vi "Part 1.vi"(11 "Input":string="#############\n#...........#\n###B#C#A#B###\n  #D#C#B#A#\n  #D#B#A#C#\n  #C#D#D#A#\n  #########") -> (3 "Output":i64=49742)   [LabVIEW 2020]
panel:
  out "Moves":string[](array[string])=["H0 -> C0", "H10 -> B0", "H9 -> B1", "H7 -> C1", "H1 -> C2", "H5 -> B2", "H3 -> B3", "H5 -> B3", "H7 -> B2", "H7 -> D0", "H7 -> B1", "H5 -> C3", "H9 -> C3", "H10 -> C2", "H10 -> D1", "H7 -> D2", "H7 -> C1", "H9 -> D3", "H5 -> D3", "H3 -> D2", "H3 -> A0", "H3 -> B0", "H7 -> A1", "H7 -> D1", "H7 -> A2", "H7 -> D0", "H5 -> A3", "H1 -> A3", "H5 -> C0", "H9 -> A2", "H10 -> A1", "H0 -> A0"]
  out "Lowest":i64=49742
  out "Solved":i32=137
  out "Paths":i32=60
  out "Counter":i32=1143083
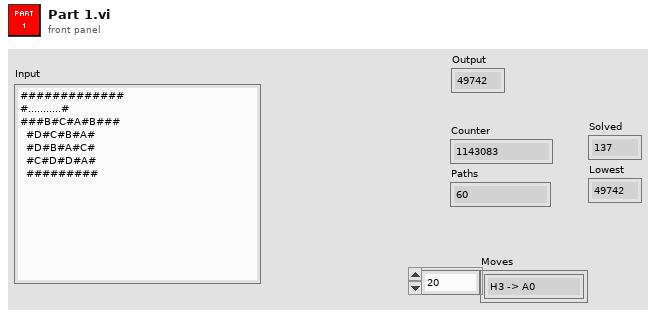
[diagram p1: front panel]
types:
  T1 = typedef "Data.ctl" = cluster{"Score":i64, "Data":cluster{"Hallway":string[], "Column A":string[], "Column B":string[], "Column C":string[], "Column D":string[]}, "Solved":bool, "Moves":string[]}
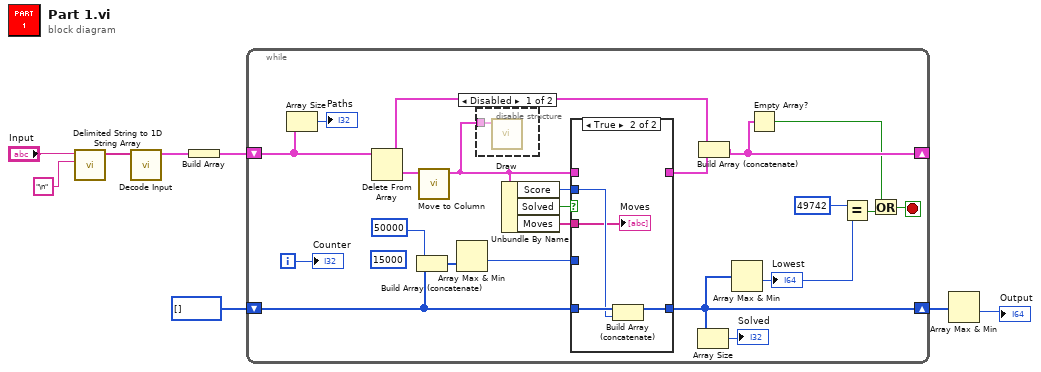
[diagram p0: block diagram]
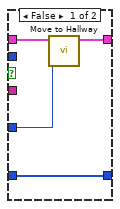
[diagram p3: hidden frame]
diagram:
  n1 = call <vilib>:"Delimited String to 1D String Array.vi"("delimiter"="\n", "delimited string"="Input") -> ("string array"=w6:string[])  [unwired: 9 in]
  n2 = call "Decode Input.vi"("Input"=w6) -> ("Data"=w1:T1)  [unwired: 10 in]
  n3 = Build Array(w1) -> (w5:T1[])
  n4 = while {
    shift-right: [w24] -> _
    shift-left: w5 -> [w18]
    shift-right: [w22] -> w3
    shift-left: i64[] [] -> [w21]
    i -> [w30]
    stop <- w10 stop-if-true
    (unwired) i64 15000 ("Max Score")
    n5 = Array Size(array=w18) -> (size(s)=→"Paths":i32)
    n6 = Delete From Array(array=w18) -> (deleted portion=w17:T1, array with subset deleted=w26:T1[])  [unwired: 2 in]
    n7 = Build Array (concatenate)(i64 50000 ("Max Score"), w21) -> (w20:i64[])
    n8 = call "Move to Column.vi"("Data In"=w17) -> ("Data Out"=w16:T1)  [unwired: 10 in]
    n9 = Array Max & Min(array=w20) -> (min value=w19:i64)  [unwired: 3 out]
    n10 = disable-structure shown="Disabled" {
      disable-tunnel: w16 -> [w31 _]
      frame Disabled {
        n11 = call "Draw.vi"("Data In"=w31) -> ()  [unwired: 11 in]
      }
      frame Enabled {
      }
    }
    n12 = Unbundle By Name(w16) -> ("Score"=w27:i64, "Solved"=w28:bool, "Moves"=w9:string[])
    n13 = case shown="True" w28 {
      tunnel: w16 -> [w35 _]
      tunnel: w27 -> [_ w38]
      tunnel: [w34 _] -> w25
      tunnel: w21 -> [w33 w39]
      tunnel: [w33 w37] -> w22
      tunnel: w19 -> [w32 _]
      tunnel: w9 -> [_ w36]
      frame False {
        n14 = call "Move to Hallway.vi"("Max Score"=w32, "Data In"=w35) -> ("Data Out"=w34:T1[])  [unwired: 9 in]
      }
      frame True {
        n15 = Build Array (concatenate)(w39, w38) -> (w37:i64[])
        "Moves" <- w36
      }
    }
    n16 = Array Size(array=w22) -> (size(s)=→"Solved":i32)
    n17 = Build Array (concatenate)(w26, w25) -> (w24:T1[])
    n18 = Array Max & Min(array=w22) -> (min value=w14:i64)  [unwired: 3 out]
    "Lowest" <- w14
    n19 = Empty Array?(array=w24) -> (empty?=w11:bool)
    n20 = Equal?(x=i64 49742, y=w14) -> (x = y?=w12:bool)
    n21 = Or(x=w11, y=w12) -> (x .or. y?=w10:bool)
    "Counter" <- w30
  }
  n22 = Array Max & Min(array=w3) -> (min value=→"Output":i64)  [unwired: 3 out]
